vi "State Machine Kernel.vi"(4 "Init?":bool, 5 "Inputs":T4 {"Kobuki Sensors"."Charger Source" items=["DISCHARGING"=0, "DOCKING_CHARGED"=2, "DOCKING_CHARGING"=6, "ADAPTER_CHARGED"=18, "ADAPTER_CHARGING"=22]; "accelerometer"."z axis (g)" format="%.3f"; "accelerometer"."y axis (g)" format="%.3f"; "accelerometer"."x axis (g)" format="%.3f"}, 7 "StateData In":T1) -> (0 "Terminated?":bool, 2 "Outputs":T3, 3 "StateData Out":T1)   [LabVIEW 2017]
uses:
  controls/Inputs.ctl
  shared/Accelerometer.ctl
  Kobuki/KobukiSensors.ctl
  Kobuki/Kobuki Bumps and WheelDrops.ctl
  Kobuki/Kobuki Buttons.ctl
  controls/Outputs.ctl
  controls/StateData.ctl
  controls/StatesEnum.ctl
panel:
  # "Electrical: charging, battery, OI mode"
  # "Sensors: bump, cliff, button, wheel drop"
  # "Motors:"
  # "Inertia"
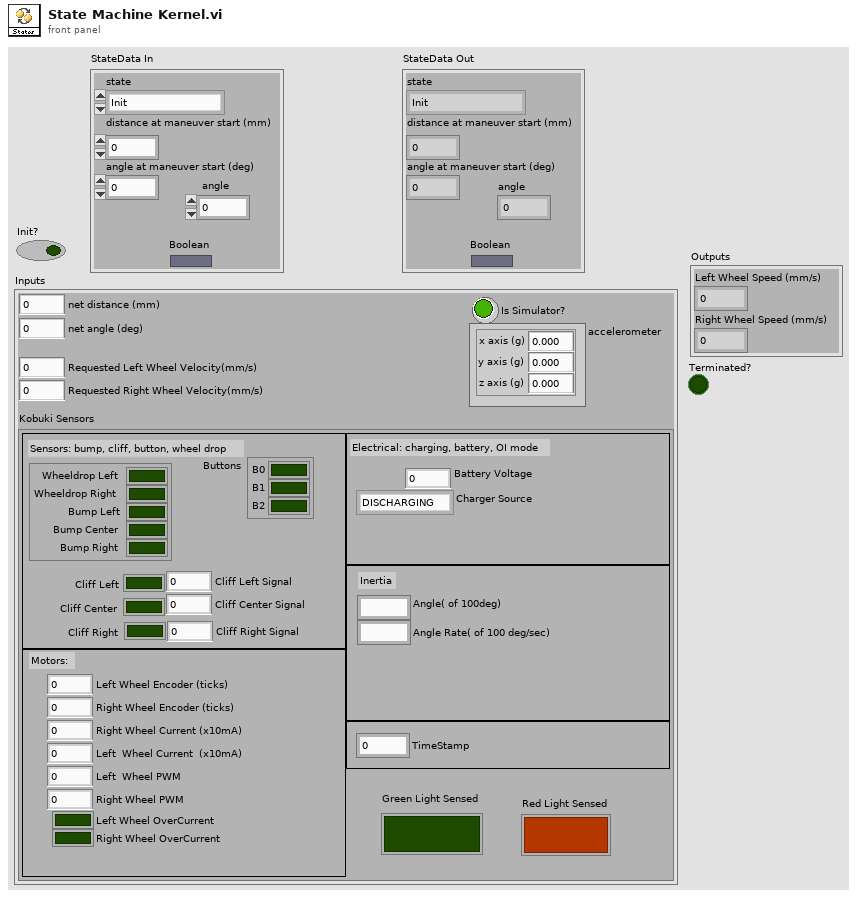
[diagram p1: front panel]
types:
  T1 = typedef "StateData.ctl" = cluster{"distance at maneuver start (mm)":i32, "angle at maneuver start (deg)":i32, "state":T2, "Boolean":bool, "angle":i32}
  T2 = typedef "StatesEnum.ctl" = enum16{"Init", "Center Cliff\n", "Pause", "Drive", "U.Turn", "L.Cliff", "R.Cliff", "Shut", "L.Bump", "R.Bump", "Red Light"}
  T3 = typedef "Outputs.ctl" = cluster{"Left Wheel Speed (mm/s)":i16, "Right Wheel Speed (mm/s)":i16}
  T4 = typedef "Inputs.ctl" = cluster{"net distance (mm)":i32, "net angle (deg)":i32, "accelerometer":T5, "Is Simulator?":bool, "Kobuki Sensors":T6, "Requested Left Wheel Velocity(mm/s)":i32, "Requested Right Wheel Velocity(mm/s)":i32, "Green Light Sensed":bool, "Red Light Sensed":bool}
  T5 = typedef "Accelerometer.ctl" = cluster{"x axis (g)":dbl, "y axis (g)":dbl, "z axis (g)":dbl}
  T6 = typedef "KobukiSensors.ctl" = cluster{"Bumps + Wheel Drops":T7, "Cliff Left":bool, "Cliff Center":bool, "Cliff Right":bool, "Cliff Left Signal":u16, "Cliff Center Signal":u16, "Cliff Right Signal":u16, "Buttons":T8, "Left Wheel Encoder (ticks)":u16, "Right Wheel Encoder (ticks) ":u16, "Left  Wheel PWM":i8, "Right Wheel PWM":i8, "Left Wheel OverCurrent":bool, "Right Wheel OverCurrent ":bool, "Right Wheel Current (x10mA)":i16, "Left  Wheel Current  (x10mA)":i16, "TimeStamp":u16, "Battery Voltage":dbl, "Angle( of 100deg)":i16, "Angle Rate( of 100 deg/sec)":i16, "Charger Source ":i8}
  T7 = typedef "Kobuki Bumps and WheelDrops.ctl" = cluster{"Wheeldrop Left":bool, "Wheeldrop Right":bool, "Bump Left":bool, "Bump Center":bool, "Bump Right":bool}
  T8 = typedef "Kobuki Buttons.ctl" = cluster{"B0":bool, "B1":bool, "B2":bool}
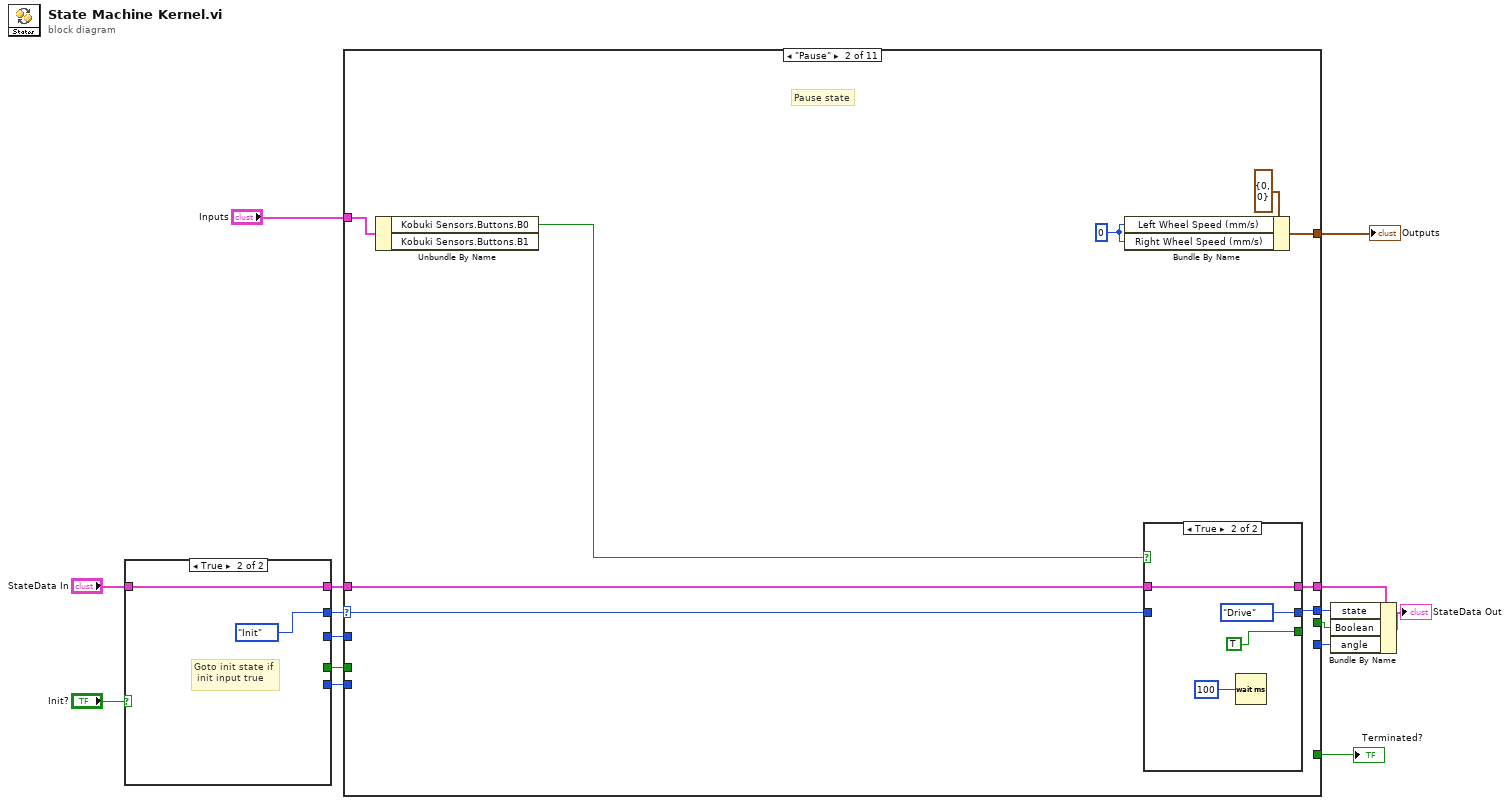
[diagram p0: block diagram]
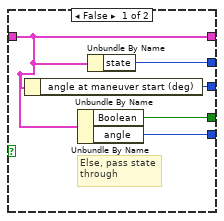
[diagram p2: hidden frame]
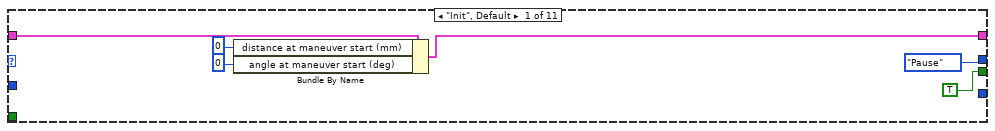
[diagram p3: hidden frame]
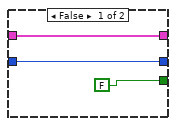
[diagram p4: hidden frame]
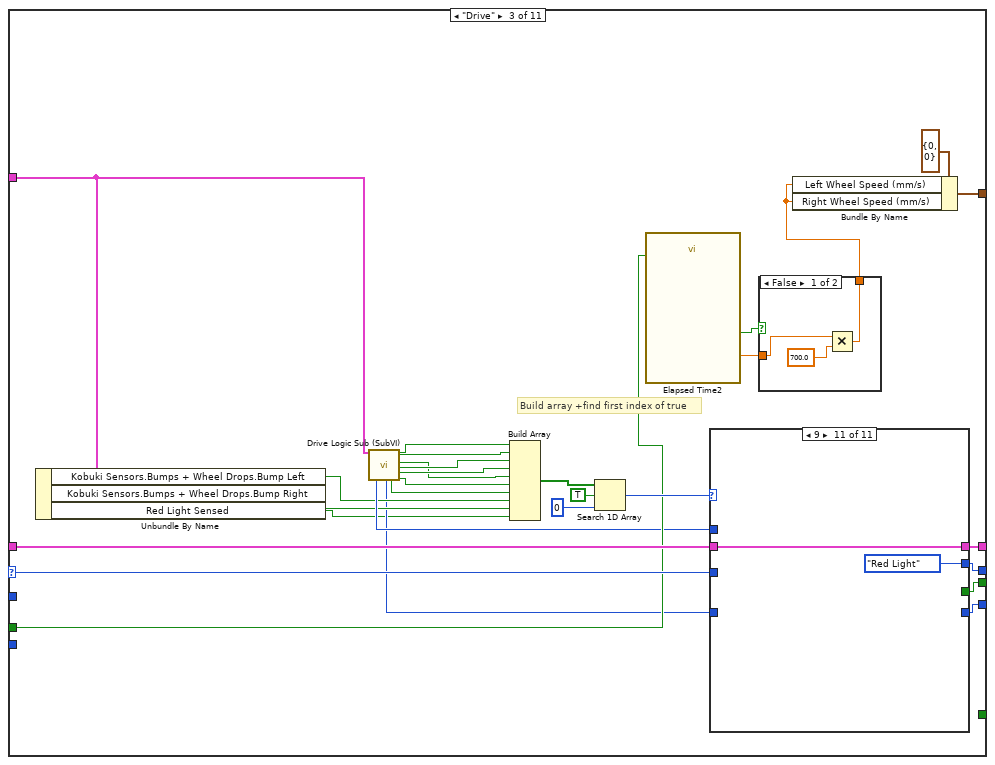
[diagram p5: hidden frame]
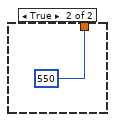
[diagram p6: hidden frame]
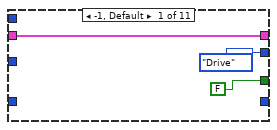
[diagram p7: hidden frame]
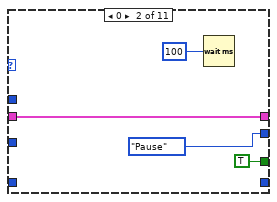
[diagram p8: hidden frame]
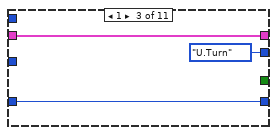
[diagram p9: hidden frame]
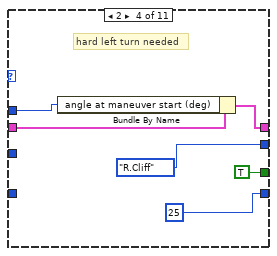
[diagram p10: hidden frame]
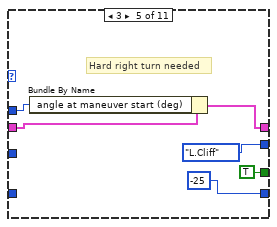
[diagram p11: hidden frame]
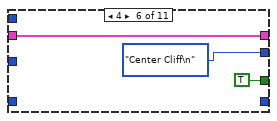
[diagram p12: hidden frame]
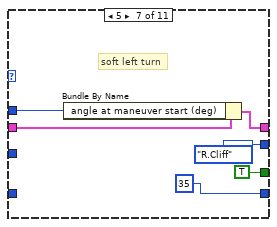
[diagram p13: hidden frame]
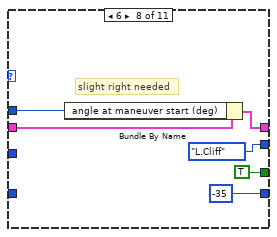
[diagram p14: hidden frame]
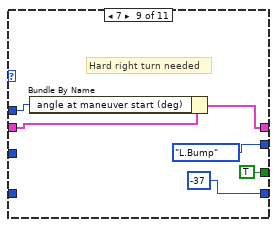
[diagram p15: hidden frame]
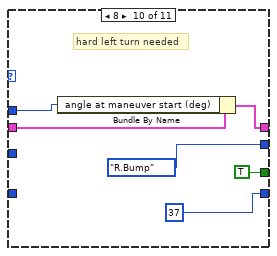
[diagram p16: hidden frame]
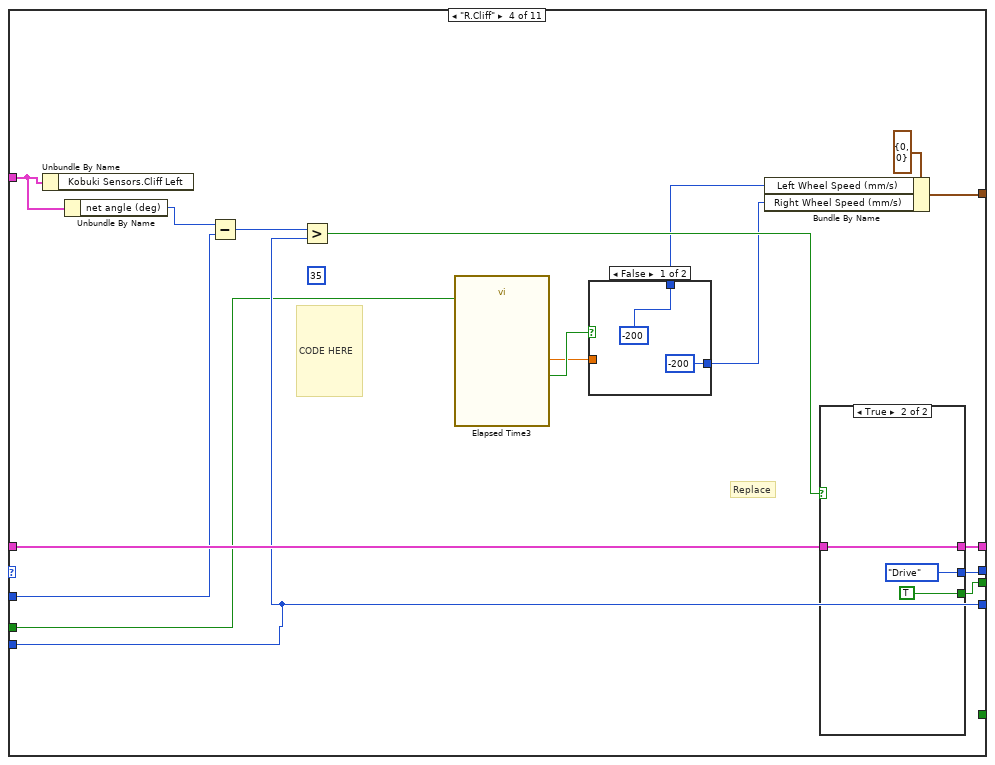
[diagram p17: hidden frame]
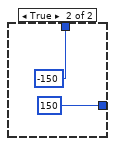
[diagram p18: hidden frame]
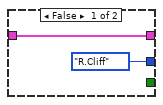
[diagram p19: hidden frame]
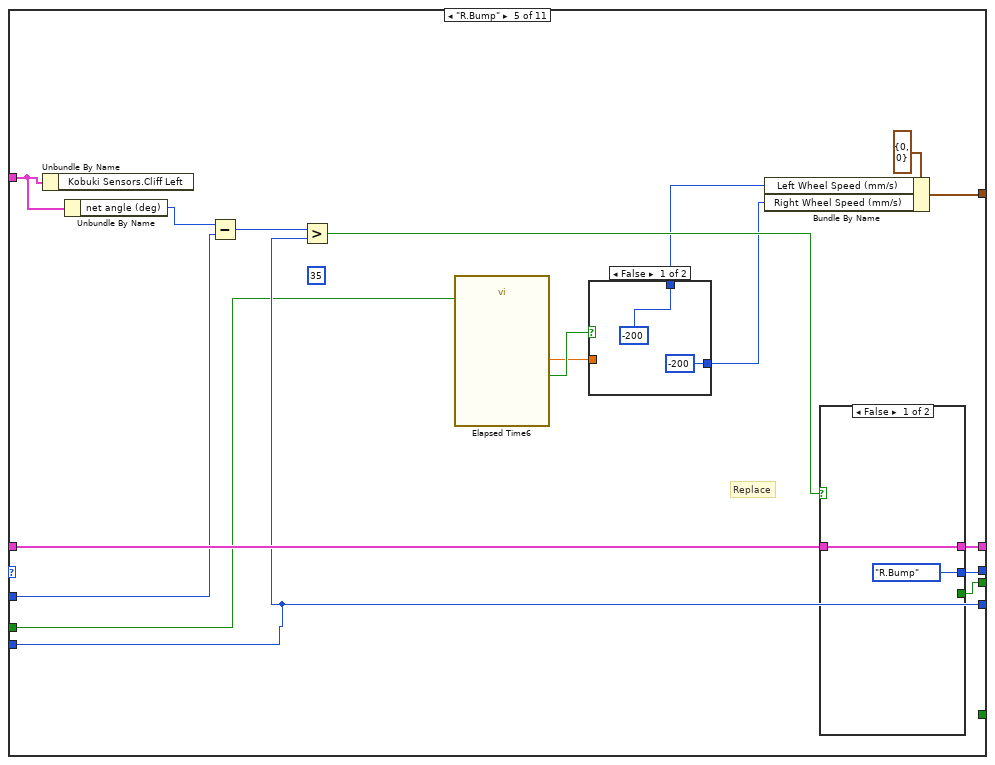
[diagram p20: hidden frame]
diagram:
  n1 = case shown="True" "Init?" {
    tunnel: [w20 StatesEnum."Init" ("StateIn")] -> w13
    tunnel: "StateData In" -> [w18 w21]
    tunnel: [w18 w21] -> w9
    tunnel: [w19 _] -> w6
    tunnel: [w17 _] -> w5
    tunnel: [w16 _] -> w2
    frame False {
      # "Else, pass state \nthrough"
      n2 = Unbundle By Name(w18) -> ("angle at maneuver start (deg)"=w19:i32)
      n3 = Unbundle By Name(w18) -> ("Boolean"=w17:bool, "angle"=w16:i32)
      n4 = Unbundle By Name(w18) -> ("state"=w20:T2)
    }
    frame True {
      # "Goto init state if\n init input true"
    }
  }
  n5 = case shown="\"Pause\"" w13 {
    selector: w13 -> [_ w33 w73 _ _ _ _ _ _ _ w306]
    tunnel: "Inputs" -> [_ w34 w49 w139 w165 w193 w222 w250 w276 w297 _]
    tunnel: [_ w37 w71 w144 w170 w196 w225 w248 w279 w291 w309] -> w11
    tunnel: [_ _ _ _ _ _ _ _ _ _ TRUE] -> w12
    tunnel: w9 -> [w28 w31 w66 w142 w168 w194 w223 w246 w277 w293 w307]
    tunnel: [w27 w30 w65 w143 w169 w195 w224 w245 w278 w292 w307] -> w8
    tunnel: w6 -> [_ _ _ w138 w164 w191 w220 _ w274 _ _]
    tunnel: w5 -> [_ _ w64 w131 w157 w183 w212 w239 _ _ _]
    tunnel: [TRUE _ w59 w135 w161 w187 w216 w244 w271 w294 _] -> w4
    tunnel: [StatesEnum."Pause" ("StateIn") w29 w60 w136 w162 w188 w217 w243 w272 w295 w306] -> w3
    tunnel: w2 -> [_ _ _ w134 w160 w186 w215 _ w264 _ _]
    tunnel: [_ _ w58 w134 w160 w186 w215 _ w264 _ _] -> w1
    frame "Init", Default {
      n6 = Bundle By Name(cluster=w28, "distance at maneuver start (mm)"=0, "angle at maneuver start (deg)"=0) -> (w27:T1)
    }
    frame "Pause" {
      w36 = i16 0 ("Left Wheel Speed (mm/s)")
      # "Pause state"
      n7 = Unbundle By Name(w34) -> ("Kobuki Sensors.Buttons.B0"=w35:bool)  [unwired: 1 out]
      n8 = Bundle By Name(cluster=T3 {"Left Wheel Speed (mm/s)"=0, "Right Wheel Speed (mm/s)"=0} ("Outputs"), "Left Wheel Speed (mm/s)"=w36, "Right Wheel Speed (mm/s)"=w36) -> (w37:T3)
      n9 = case shown="True" w35 {
        tunnel: w33 -> [w40 _]
        tunnel: [w40 StatesEnum."Drive" ("StateIn")] -> w29
        tunnel: w31 -> [w39 w42]
        tunnel: [w39 w42] -> w30
        tunnel: [FALSE TRUE] -> _
        frame False {
        }
        frame True {
          n10 = Wait (ms)(milliseconds to wait=u32 100) -> ()  [unwired: 1 out]
        }
      }
    }
    frame "Drive" {
      # "Build array +find first index of true"
      n11 = Unbundle By Name(w49) -> ("Kobuki Sensors.Bumps + Wheel Drops.Bump Left"=w48:bool, "Kobuki Sensors.Bumps + Wheel Drops.Bump Right"=w47:bool, "Red Light Sensed"=w45:bool)
      n12 = call "Drive Logic Sub (SubVI).vi"("Inputs"=w49) -> ("net angle (deg)"=w57:i32, "U-turn Angle"=w46:i32, "Soft Left Cliff"=w50:bool, "Pause"=w56:bool, "U.Turn"=w55:bool, "Center"=w52:bool, "Hard Right Cliff"=w54:bool, "Hard Left Cliff"=w53:bool, "Soft Right Cliff"=w51:bool)  [unwired: 10 in]
      n13 = Build Array(w56, w55, w54, w53, w52, w51, w50, w48, w47, w45) -> (w70:bool[])
      n14 = Search 1D Array(1D array=w70, element=TRUE, start index (0)=0) -> (index of element=w67:i32)
      n15 = call "Elapsed Time2"("Reset"=w64) -> ("Elapsed Time (s)"=w62:dbl, "Time has Elapsed"=w63:bool)  [unwired: 11 in, 6 out]
      n16 = case shown="9" w67 {
        tunnel: w73 -> [_ _ _ _ _ _ _ _ _ _ _]
        tunnel: w66 -> [w80 w83 w87 w89 w96 w101 w108 w114 w117 w122 w127]
        tunnel: [w80 w83 w87 w88 w95 w101 w107 w112 w116 w121 w127] -> w65
        tunnel: w57 -> [_ _ _ w90 w94 _ w106 w113 w115 w123 _]
        tunnel: [FALSE TRUE _ TRUE TRUE TRUE TRUE TRUE TRUE TRUE _] -> w59
        tunnel: [StatesEnum."Drive" ("StateIn") StatesEnum."Pause" ("StateIn") StatesEnum."U.Turn" ("StateIn") StatesEnum."R.Cliff" ("StateIn") StatesEnum."L.Cliff" ("StateIn") StatesEnum."Center Cliff\n" ("StateIn") StatesEnum."R.Cliff" ("StateIn") StatesEnum."L.Cliff" ("StateIn") StatesEnum."L.Bump" ("StateIn") StatesEnum."R.Bump" ("StateIn") StatesEnum."Red Light" ("StateIn")] -> w60
        tunnel: [_ _ w85 25 ("angle") -25 ("angle") _ 35 ("angle") -35 ("angle") -37 ("angle") 37 ("angle") _] -> w58
        tunnel: w46 -> [_ _ w85 _ _ _ _ _ _ _ _]
        frame -1, Default {
        }
        frame 0 {
          n17 = Wait (ms)(milliseconds to wait=u32 100) -> ()  [unwired: 1 out]
        }
        frame 1 {
        }
        frame 2 {
          # "hard left turn needed"
          n18 = Bundle By Name(cluster=w89, "angle at maneuver start (deg)"=w90) -> (w88:T1)
        }
        frame 3 {
          # "Hard right turn needed"
          n19 = Bundle By Name(cluster=w96, "angle at maneuver start (deg)"=w94) -> (w95:T1)
        }
        frame 4 {
        }
        frame 5 {
          # "soft left turn"
          n20 = Bundle By Name(cluster=w108, "angle at maneuver start (deg)"=w106) -> (w107:T1)
        }
        frame 6 {
          # "slight right needed"
          n21 = Bundle By Name(cluster=w114, "angle at maneuver start (deg)"=w113) -> (w112:T1)
        }
        frame 7 {
          # "Hard right turn needed"
          n22 = Bundle By Name(cluster=w117, "angle at maneuver start (deg)"=w115) -> (w116:T1)
        }
        frame 8 {
          # "hard left turn needed"
          n23 = Bundle By Name(cluster=w122, "angle at maneuver start (deg)"=w123) -> (w121:T1)
        }
        frame 9 {
        }
      }
      n24 = case shown="False" w63 {
        tunnel: w62 -> [w75 _]
        tunnel: [w74 550] -> w61
        frame False {
          n25 = Multiply(x=w75, y=700.0) -> (x*y=w74:dbl)
        }
        frame True {
        }
      }
      n26 = Bundle By Name(cluster=T3 {"Left Wheel Speed (mm/s)"=0, "Right Wheel Speed (mm/s)"=0} ("Outputs"), "Left Wheel Speed (mm/s)"=w61, "Right Wheel Speed (mm/s)"=w61) -> (w71:T3)
    }
    frame "R.Cliff" {
      (unwired) 35 ("y")
      # "Replace"
      # "CODE HERE"
      n27 = Unbundle By Name(w139) -> ()  [unwired: 1 out]
      n28 = Unbundle By Name(w139) -> ("net angle (deg)"=w140:i32)
      n29 = Subtract(x=w140, y=w138) -> (x-y=w141:i32)
      n30 = Greater?(x=w141, y=w134) -> (0:w137:bool)
      n31 = call "Elapsed Time3"("Reset"=w131) -> ("Elapsed Time (s)"=w132:dbl, "Time has Elapsed"=w133:bool)  [unwired: 11 in, 6 out]
      n32 = case shown="False" w133 {
        tunnel: w132 -> [_ _]
        tunnel: [-200 150] -> w129
        tunnel: [-200 -150] -> w130
        frame False {
        }
        frame True {
        }
      }
      n33 = Bundle By Name(cluster=T3 {"Left Wheel Speed (mm/s)"=0, "Right Wheel Speed (mm/s)"=0} ("Outputs"), "Left Wheel Speed (mm/s)"=w130, "Right Wheel Speed (mm/s)"=w129) -> (w144:T3)
      n34 = case shown="True" w137 {
        tunnel: [StatesEnum."R.Cliff" ("StateIn") StatesEnum."Drive" ("StateIn")] -> w136
        tunnel: w142 -> [w150 w153]
        tunnel: [w150 w153] -> w143
        tunnel: [_ TRUE ("Boolean")] -> w135
        frame False {
        }
        frame True {
        }
      }
    }
    frame "R.Bump" {
      (unwired) 35 ("y")
      # "Replace"
      n35 = Unbundle By Name(w165) -> ()  [unwired: 1 out]
      n36 = Unbundle By Name(w165) -> ("net angle (deg)"=w166:i32)
      n37 = Subtract(x=w166, y=w164) -> (x-y=w167:i32)
      n38 = Greater?(x=w167, y=w160) -> (0:w163:bool)
      n39 = call "Elapsed Time6"("Reset"=w157) -> ("Elapsed Time (s)"=w158:dbl, "Time has Elapsed"=w159:bool)  [unwired: 11 in, 6 out]
      n40 = case shown="False" w159 {
        tunnel: w158 -> [_ _]
        tunnel: [-200 150] -> w155
        tunnel: [-200 -150] -> w156
        frame False {
        }
        frame True {
        }
      }
      n41 = Bundle By Name(cluster=T3 {"Left Wheel Speed (mm/s)"=0, "Right Wheel Speed (mm/s)"=0} ("Outputs"), "Left Wheel Speed (mm/s)"=w156, "Right Wheel Speed (mm/s)"=w155) -> (w170:T3)
      n42 = case shown="False" w163 {
        tunnel: [StatesEnum."R.Bump" ("StateIn") StatesEnum."Drive" ("StateIn")] -> w162
        tunnel: w168 -> [w176 w179]
        tunnel: [w176 w179] -> w169
        tunnel: [_ TRUE ("Boolean")] -> w161
        frame False {
        }
        frame True {
        }
      }
    }
    frame "L.Cliff" {
      (unwired) -35 ("y")
      n43 = Unbundle By Name(w193) -> ()  [unwired: 1 out]
      n44 = Unbundle By Name(w193) -> ("net angle (deg)"=w192:i32)
      n45 = Subtract(x=w192, y=w191) -> (x-y=w190:i32)
      n46 = Less?(x=w190, y=w186) -> (x < y?=w189:bool)
      n47 = call "Elapsed Time"("Reset"=w183) -> ("Elapsed Time (s)"=w184:dbl, "Time has Elapsed"=w185:bool)  [unwired: 11 in, 6 out]
      n48 = case shown="True" w185 {
        tunnel: w184 -> [w200 _]
        tunnel: [w198 i16 -150] -> w182
        tunnel: [w198 i16 150] -> w181
        frame False {
          w198 = i16 -200 ("16bit integer")
          n49 = Multiply(x=w200, y=-700.0) -> (x*y=w199:dbl)
          n50 = To Word Integer(number=w199) -> ()  [unwired: 1 out]
        }
        frame True {
        }
      }
      n51 = Bundle By Name(cluster=T3 {"Left Wheel Speed (mm/s)"=0, "Right Wheel Speed (mm/s)"=0} ("Outputs"), "Left Wheel Speed (mm/s)"=w181, "Right Wheel Speed (mm/s)"=w182) -> (w196:T3)
      n52 = case shown="False" w189 {
        tunnel: [StatesEnum."L.Cliff" ("StateIn") StatesEnum."Drive" ("StateIn")] -> w188
        tunnel: w194 -> [w205 w208]
        tunnel: [w205 w208] -> w195
        tunnel: [FALSE ("Boolean") TRUE ("Boolean")] -> w187
        frame False {
        }
        frame True {
        }
      }
    }
    frame "L.Bump" {
      (unwired) -35 ("y")
      n53 = Unbundle By Name(w222) -> ()  [unwired: 1 out]
      n54 = Unbundle By Name(w222) -> ("net angle (deg)"=w221:i32)
      n55 = Subtract(x=w221, y=w220) -> (x-y=w219:i32)
      n56 = Less?(x=w219, y=w215) -> (x < y?=w218:bool)
      n57 = call "Elapsed Time5"("Reset"=w212) -> ("Elapsed Time (s)"=w213:dbl, "Time has Elapsed"=w214:bool)  [unwired: 11 in, 6 out]
      n58 = case shown="True" w214 {
        tunnel: w213 -> [w229 _]
        tunnel: [w227 i16 -150] -> w211
        tunnel: [w227 i16 150] -> w210
        frame False {
          w227 = i16 -200 ("16bit integer")
          n59 = Multiply(x=w229, y=-700.0) -> (x*y=w228:dbl)
          n60 = To Word Integer(number=w228) -> ()  [unwired: 1 out]
        }
        frame True {
        }
      }
      n61 = Bundle By Name(cluster=T3 {"Left Wheel Speed (mm/s)"=0, "Right Wheel Speed (mm/s)"=0} ("Outputs"), "Left Wheel Speed (mm/s)"=w210, "Right Wheel Speed (mm/s)"=w211) -> (w225:T3)
      n62 = case shown="True" w218 {
        tunnel: [StatesEnum."L.Bump" ("StateIn") StatesEnum."Drive" ("StateIn")] -> w217
        tunnel: w223 -> [w234 w237]
        tunnel: [w234 w237] -> w224
        tunnel: [FALSE ("Boolean") TRUE ("Boolean")] -> w216
        frame False {
        }
        frame True {
        }
      }
    }
    frame "Center Cliff\n" {
      w247 = i16 -150 ("Left Wheel Speed (mm/s)")
      n63 = Unbundle By Name(w250) -> ()  [unwired: 5 out]
      n64 = call "Elapsed Time4"("Reset"=w239) -> ("Elapsed Time (s)"=w241:dbl, "Time has Elapsed"=w242:bool)  [unwired: 11 in, 6 out]
      n65 = case shown="True" w242 {
        tunnel: w241 -> [_ _]
        tunnel: [-200 150] -> _
        tunnel: [-200 -150] -> _
        tunnel: [FALSE TRUE] -> w240
        frame False {
        }
        frame True {
        }
      }
      n66 = case shown="False" w240 {
        tunnel: w246 -> [w258 w262]
        tunnel: [w258 w262] -> w245
        tunnel: [FALSE ("Boolean") TRUE ("Boolean")] -> w244
        tunnel: [StatesEnum."Center Cliff\n" ("StateIn") StatesEnum."Drive" ("StateIn")] -> w243
        frame False {
        }
        frame True {
        }
      }
      n67 = Bundle By Name(cluster=T3 {"Left Wheel Speed (mm/s)"=0, "Right Wheel Speed (mm/s)"=0} ("Outputs"), "Left Wheel Speed (mm/s)"=w247, "Right Wheel Speed (mm/s)"=w247) -> (w248:T3)
    }
    frame "U.Turn" {
      n68 = Unbundle By Name(w276) -> ("net angle (deg)"=w275:i32)
      n69 = Subtract(x=w275, y=w274) -> (x-y=w266:i32)
      n70 = Absolute Value(x=w266) -> (abs(x)=w265:i32)
      n71 = Absolute Value(x=w264) -> (abs(x)=w263:i32)
      n72 = Greater?(x=w264, y=0) -> (0:w267:bool)
      n73 = Greater?(x=w265, y=w263) -> (0:w273:bool)
      n74 = case shown="False" w267 {
        tunnel: [i16 -150 i16 150] -> w270
        tunnel: [i16 150 i16 -150] -> w269
        frame False {
        }
        frame True {
        }
      }
      n75 = Bundle By Name(cluster=T3 {"Left Wheel Speed (mm/s)"=0, "Right Wheel Speed (mm/s)"=0} ("Outputs"), "Left Wheel Speed (mm/s)"=w269, "Right Wheel Speed (mm/s)"=w270) -> (w279:T3)
      n76 = case shown="False" w273 {
        tunnel: [StatesEnum."U.Turn" ("StateIn") StatesEnum."Drive" ("StateIn")] -> w272
        tunnel: w277 -> [w286 w289]
        tunnel: [w286 w289] -> w278
        tunnel: [FALSE ("Boolean") TRUE ("Boolean")] -> w271
        frame False {
        }
        frame True {
        }
      }
    }
    frame "Red Light" {
      w291 = T3 {"Left Wheel Speed (mm/s)"=0, "Right Wheel Speed (mm/s)"=0} ("Outputs")
      # "Stop until green light is sensed. Anything else necessary?"
      n77 = Unbundle By Name(w297) -> ("Green Light Sensed"=w296:bool)
      n78 = Bundle By Name(cluster=w291, "Left Wheel Speed (mm/s)"=i16 0, "Right Wheel Speed (mm/s)"=i16 0) -> ()  [unwired: 1 out]
      n79 = case shown="False" w296 {
        tunnel: [StatesEnum."Red Light" ("StateIn") StatesEnum."Drive" ("StateIn")] -> w295
        tunnel: w293 -> [w301 w304]
        tunnel: [w301 w304] -> w292
        tunnel: [FALSE ("Boolean") TRUE ("Boolean")] -> w294
        frame False {
        }
        frame True {
        }
      }
    }
    frame "Shut" {
      w310 = i16 0 ("Left Wheel Speed (mm/s)")
      # "Shutdown"
      n80 = Bundle By Name(cluster=T3 {"Left Wheel Speed (mm/s)"=0, "Right Wheel Speed (mm/s)"=0} ("Outputs"), "Left Wheel Speed (mm/s)"=w310, "Right Wheel Speed (mm/s)"=w310) -> (w309:T3)
    }
  }
  "Terminated?" <- w12
  "Outputs" <- w11
  n81 = Bundle By Name(cluster=w8, "state"=w3, "Boolean"=w4, "angle"=w1) -> (→"StateData Out":T1)
